vi "ChaxuConfigDlg.vi"(8 "error in":errorcluster) -> (0 "error out":errorcluster)   [LabVIEW 2014, in "ChaxuConfig.lvlib"]
uses:
  ChaxuConfig.lvlib
  <vilib>/Utility/file.llb/Write To Spreadsheet File (string).vi
  DataBase/DataBase.lvlib
  DetectElecrodes/DetectElectros.lvlib
panel:
  in  "表格导出":bool
  out "new file path (Not A Path if cancelled) 2":path caption="新建文件路径（取消时为非法路径）"
  in  "选项卡控件":enum32{"检测电极配置信息", "供电电极配置信息"}(tab)
  in  "配置信息":i32(listbox)
  in  "供电电极配置信息":i32(listbox)
  out "new file path (Not A Path if cancelled)":path caption="新建文件路径（取消时为非法路径）"
  in  "电极信息选择":u16(ring) items=["检测电极配置", "供电电极配置"]
  in  "表格导出":bool
  in  "查询":bool
  in  "退出":bool
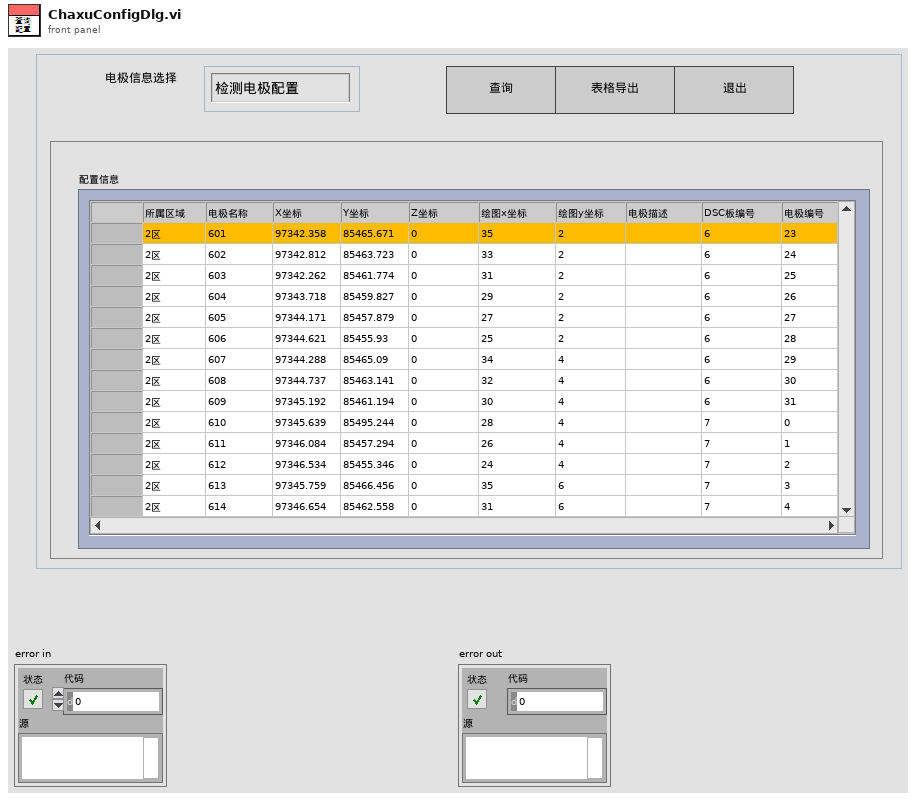
[diagram p1: front panel]
types:
  T1 = enum32{"invalid app kind", "Development System", "Run Time System", "Student Edition", "Embedded LabVIEW", "Evaluation", "Custom"}
  T2 = enum32{"Invalid", "Standard", "Closed", "Hidden", "Minimized", "Maximized"}
  T3 = cluster{"Core":cluster{"Current VI Reference":refnum<vi>, "Close Panel on Exit?":bool}, "Your Boolean data":bool, "Your string data":string, "电极信息":string[][]}
  T4 = cluster{"Current VI Reference":refnum<vi>, "Close Panel on Exit?":bool}
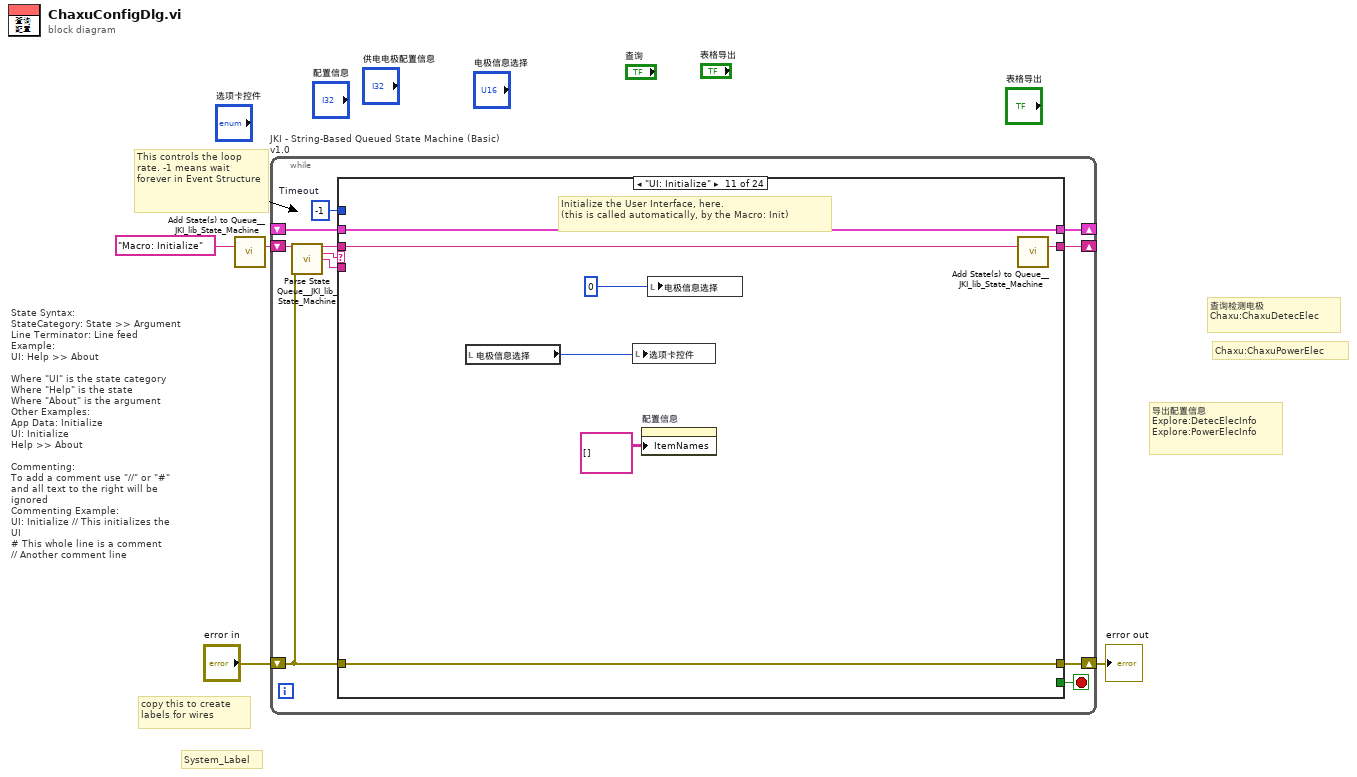
[diagram p0: block diagram]
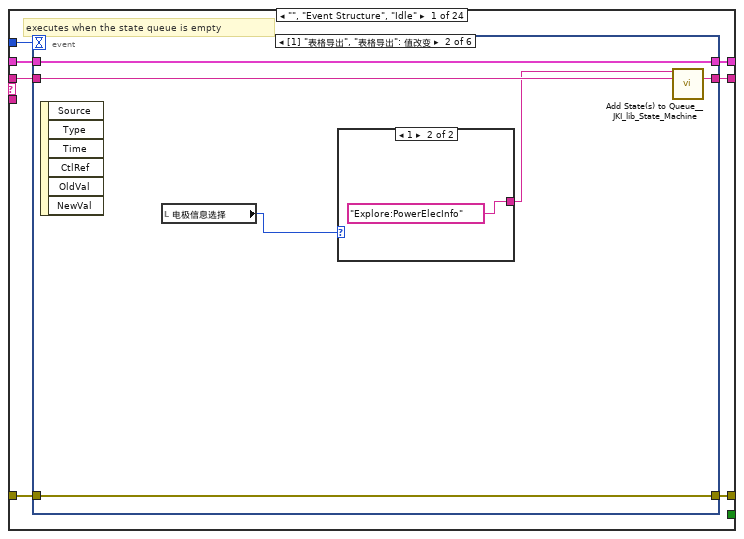
[diagram p2: hidden frame]
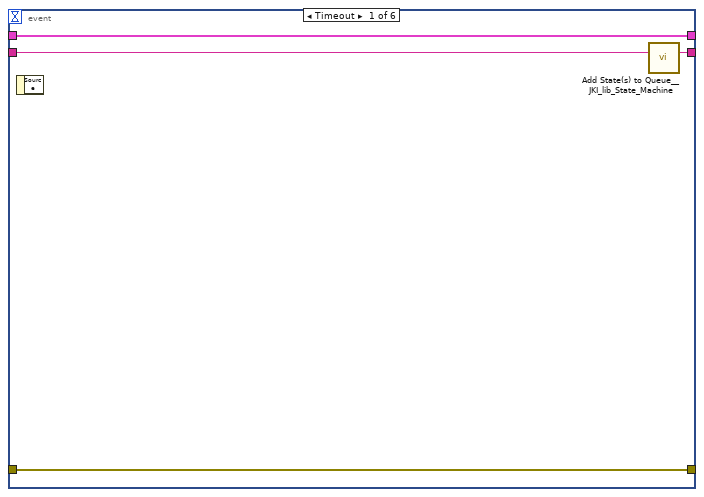
[diagram p3: hidden frame]
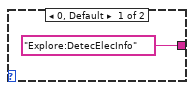
[diagram p4: hidden frame]
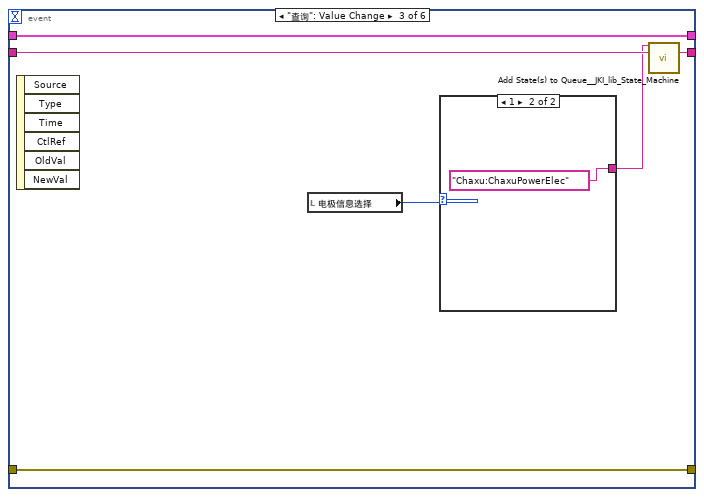
[diagram p5: hidden frame]
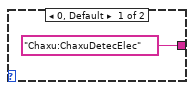
[diagram p6: hidden frame]
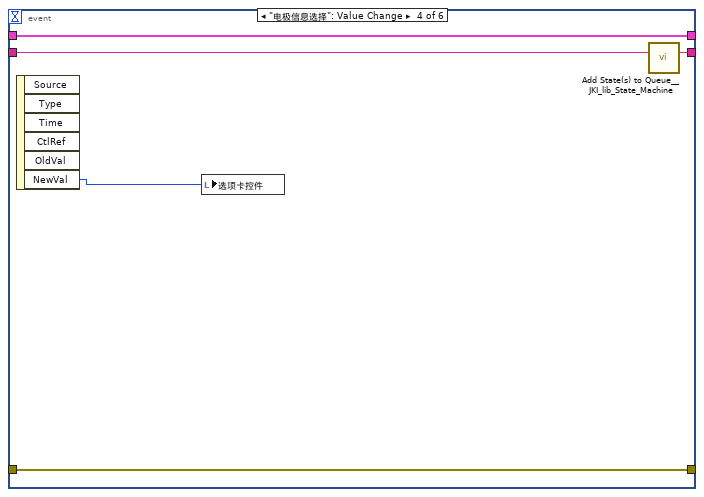
[diagram p7: hidden frame]
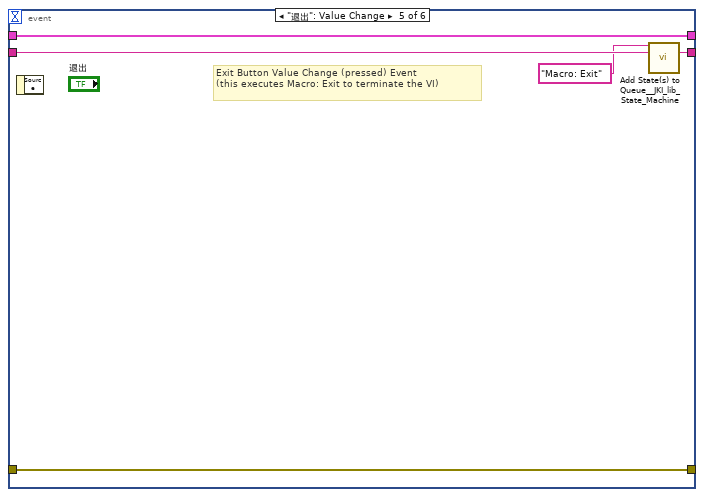
[diagram p8: hidden frame]
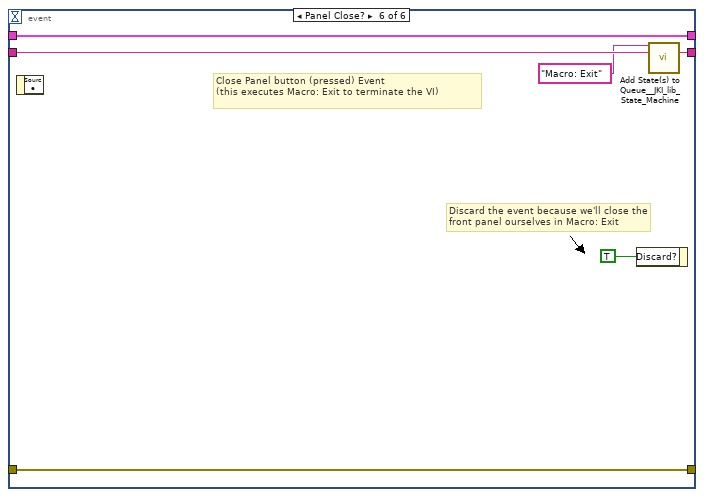
[diagram p9: hidden frame]
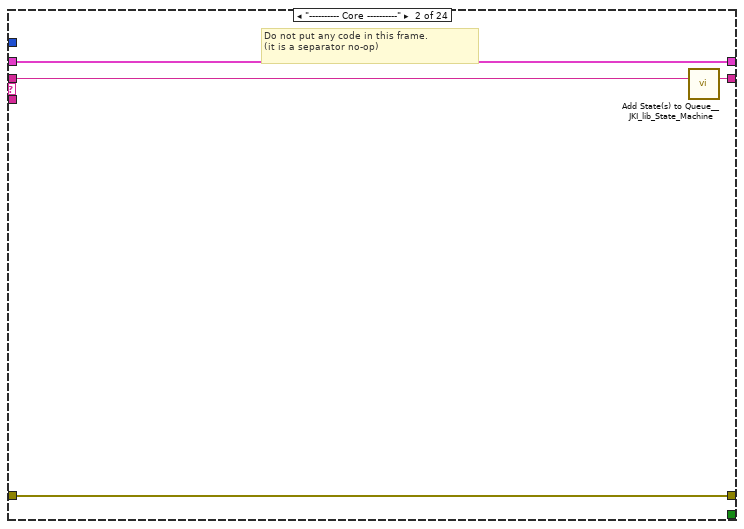
[diagram p10: hidden frame]
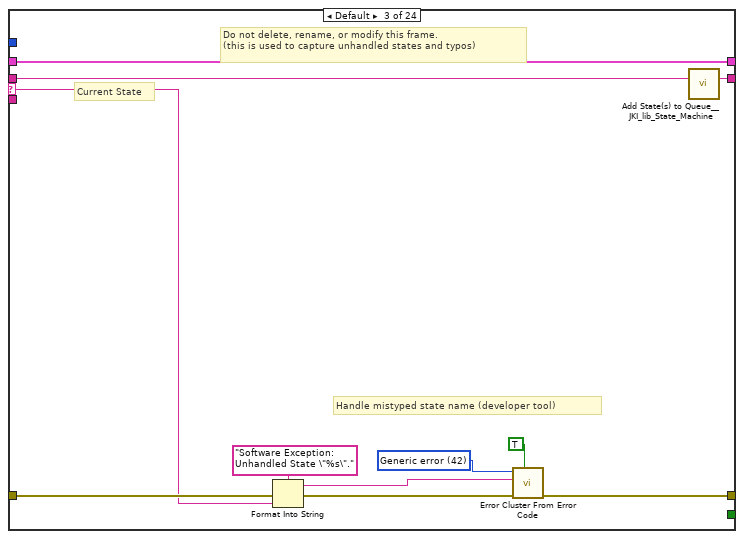
[diagram p11: hidden frame]
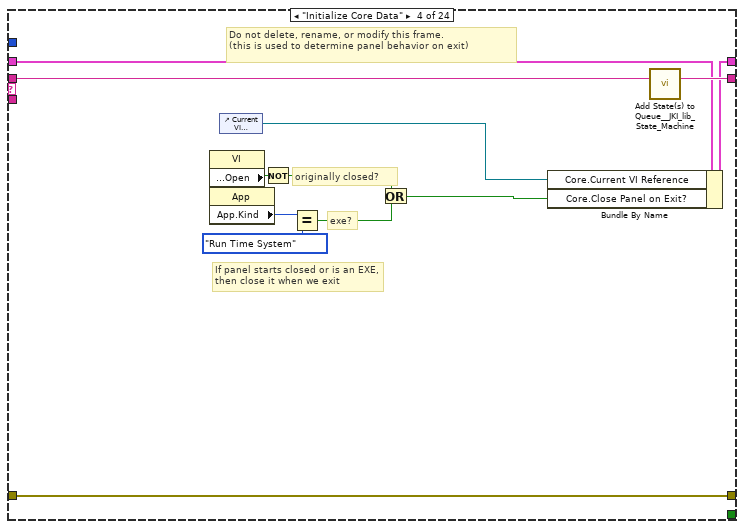
[diagram p12: hidden frame]
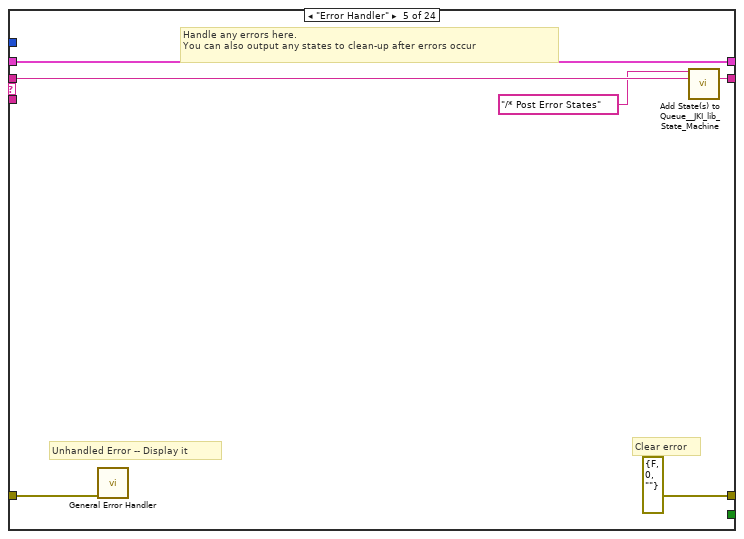
[diagram p13: hidden frame]
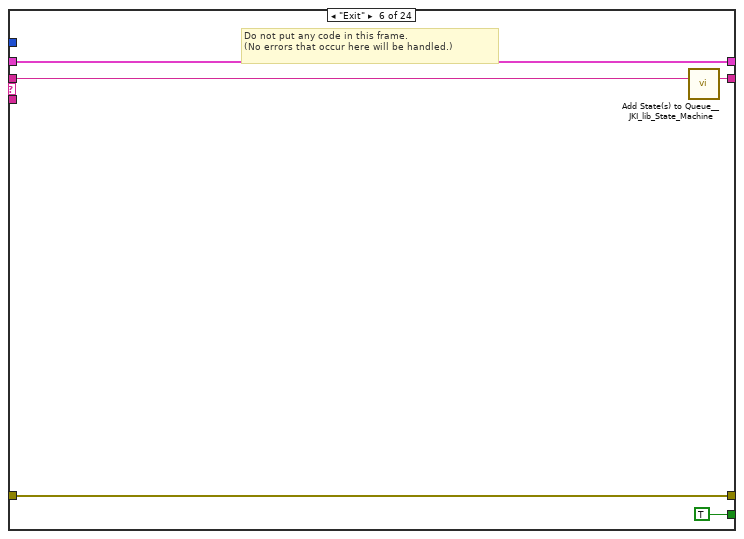
[diagram p14: hidden frame]
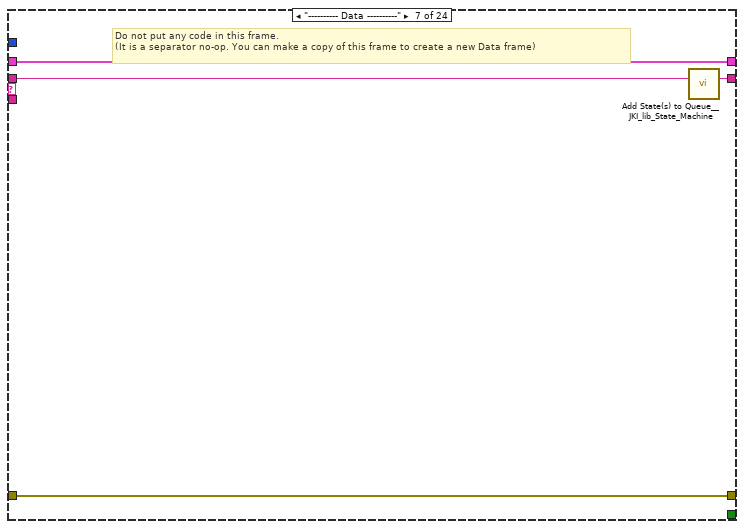
[diagram p15: hidden frame]
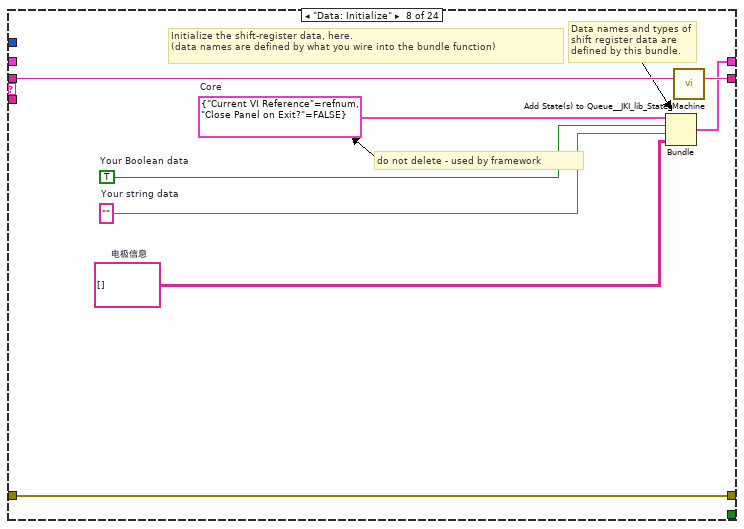
[diagram p16: hidden frame]
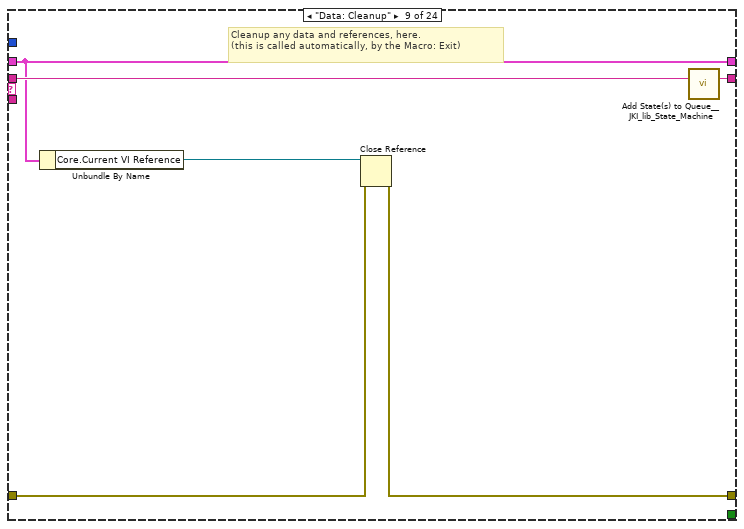
[diagram p17: hidden frame]
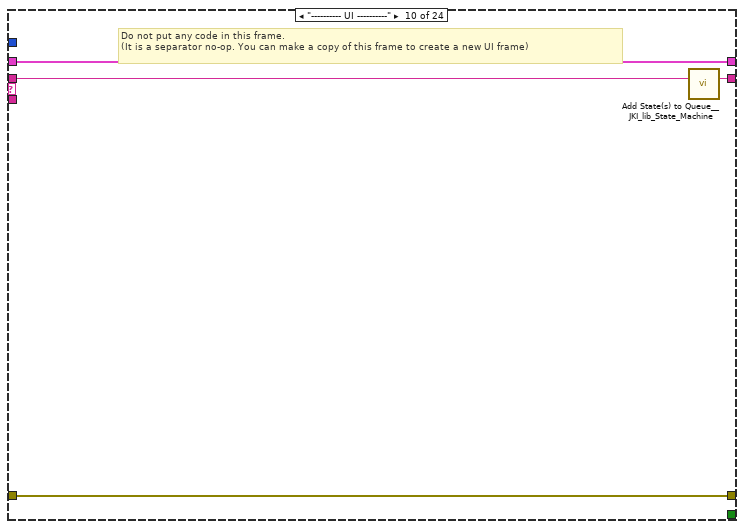
[diagram p18: hidden frame]
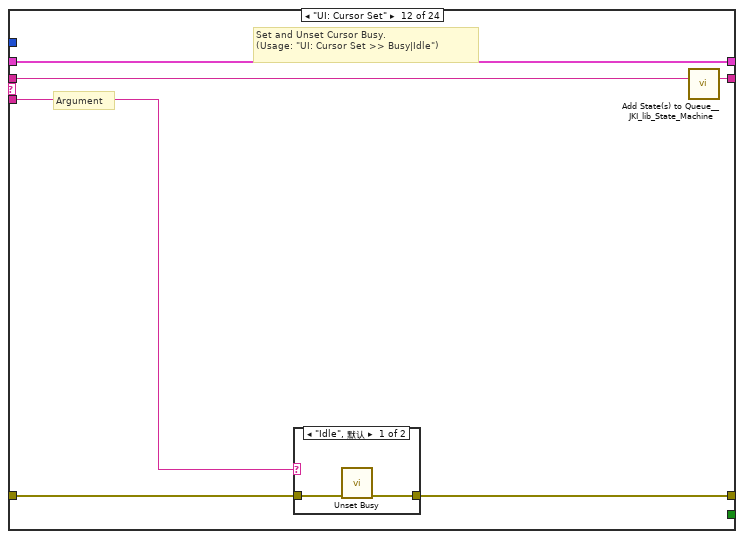
[diagram p19: hidden frame]
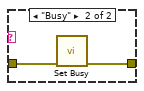
[diagram p20: hidden frame]
diagram:
  # "导出配置信息\nExplore:DetecElecInfo\nExplore:PowerElecInfo"
  # "Chaxu:ChaxuPowerElec"
  # "查询检测电极\nChaxu:ChaxuDetecElec"
  # "State Syntax:\nStateCategory: State >> Argument\nLine Terminator: Line feed\nExample:\nUI: Help >> About\n\nWhere \"UI\" is the state category\nWhere \"Help\" is the state\nWhere \"About\" is the argument\nOther Examples:\nApp Data: Initialize\nUI: Initialize\nHelp >> About\n\nCommenting:\nTo add a comment use \"//\" or \"#\" and all text to the right will be ignored\nCommenting Example:\nUI: Initialize // This initializes the UI\n# This whole line is a comment\n// Another comment line"
  # "copy this to create labels for wires"
  # "This controls the loop rate. -1 means wait forever in Event Structure"
  # "System_Label"
  n1 = call <vilib>:"Add State(s) to Queue__JKI_lib_State_Machine.vi"("State(s) in (\"\")"="Macro: Initialize") -> ("States Out"=w4:string)  [unwired: 14 in]
  n2 = while "JKI - String-Based Queued State Machine (Basic) v1.0" {
    shift-right: [w8] -> _
    shift-left: _ -> [w7]
    shift-right: [w11] -> w2
    shift-left: "error in" -> [w5]
    shift-right: [w10] -> _
    shift-left: w4 -> [w12]
    stop <- w9 stop-if-true
    w6 = -1  # Timeout
    n3 = call <vilib>:"Parse State Queue__JKI_lib_State_Machine.vi"("State Queue"=w12, "Error In (no error)"=w5) -> ("Remaining States"=w14:string, "Current State"=w15:string, "Arguments"=w13:string)  [unwired: 11 in]
    n4 = case shown="\"UI: Initialize\"" w15 {
      selector: w15 -> [_ _ w63 _ _ _ _ _ _ _ _ _ _ _ _ _ _ _ _ _ _ _ _ _]
      tunnel: w14 -> [w22 w62 w67 w85 w91 w96 w100 w108 w114 w118 w125 w131 w142 w168 w173 w183 w187 w191 w195 w200 w216 w231 w248 w265]
      tunnel: w13 -> [_ _ _ _ _ _ _ _ _ _ _ w126 w136 _ _ _ _ _ _ _ _ _ _ _]
      tunnel: w7 -> [w20 w59 w65 w76 w88 w94 w97 _ w109 w115 w123 w129 w138 w165 w170 w180 w184 w188 w192 w197 w213 w228 w233 w250]
      tunnel: [w19 w60 w69 w82 errorcluster {"status"=FALSE, "code"=0, "source"=""} ("error out") w93 w98 w105 w110 w116 w122 w127 w139 w166 w171 w181 w185 w189 w193 w198 w214 w229 w246 w263] -> w11
      tunnel: w5 -> [w18 w60 w68 w82 w87 w93 w98 w105 w111 w116 w122 w128 w140 w166 w171 w181 w185 w189 w193 w198 w214 w229 w246 w263]
      tunnel: [w21 w61 w66 w84 w90 w95 w99 w107 w113 w117 w124 w130 w141 w167 w172 w182 w186 w190 w194 w199 w215 w230 w247 w264] -> w10
      tunnel: [_ _ _ _ _ TRUE _ _ _ _ _ _ _ _ _ _ _ _ _ _ _ _ _ _] -> w9
      tunnel: [w17 w59 w65 w83 w88 w94 w97 w106 w109 w115 w123 w129 w138 w165 w170 w180 w184 w188 w192 w197 w213 w228 w232 w249] -> w8
      tunnel: w6 -> [w16 _ _ _ _ _ _ _ _ _ _ _ _ _ _ _ _ _ _ _ _ _ _ _]
      frame "", "Event Structure", "Idle" {
        # "executes when the state queue is empty"
        n5 = event shown="[1] \"表格导出\", \"表格导出\": 值改变" {
          selector: _ -> [_ _ _ _ _ _]
          dyn-events: _ -> [_ _ _ _ _ _]
          timeout: w16 -> [_ _ _ _ _ _]
          tunnel: w22 -> [w26 w32 w40 w47 w52 w58]
          tunnel: [w25 w31 w39 w46 w51 w57] -> w21
          tunnel: w20 -> [w23 w29 w37 w44 w49 w55]
          tunnel: [w24 w30 w38 w45 w50 w56] -> w19
          tunnel: w18 -> [w24 w30 w38 w45 w50 w56]
          tunnel: [w23 w29 w37 w44 w49 w55] -> w17
          event Timeout {
            n6 = event-data() -> ()  [unwired: 1 in, 1 out]
            n7 = call <vilib>:"Add State(s) to Queue__JKI_lib_State_Machine.vi"("State(s) in (\"\")"=w26) -> ("States Out"=w25:string)  [unwired: 14 in]
          }
          event "表格导出", "表格导出": Value Change {
            n8 = event-data() -> ()  [unwired: 1 in, 6 out]
            n9 = local read "电极信息选择"() -> (w27:u16)
            n10 = case shown="1" w27 {
              tunnel: ["Explore:DetecElecInfo" "Explore:PowerElecInfo"] -> w28
              frame 0, Default {
              }
              frame 1 {
              }
            }
            n11 = call <vilib>:"Add State(s) to Queue__JKI_lib_State_Machine.vi"("State(s) in Front (\"\")"=w28, "State(s) in (\"\")"=w32) -> ("States Out"=w31:string)  [unwired: 13 in]
          }
          event "查询": Value Change {
            n12 = event-data() -> ()  [unwired: 1 in, 6 out]
            n13 = local read "电极信息选择"() -> (w36:u16)
            n14 = case shown="1" w36 {
              tunnel: ["Chaxu:ChaxuDetecElec" "Chaxu:ChaxuPowerElec"] -> w35
              frame 0, Default {
              }
              frame 1 {
              }
            }
            n15 = call <vilib>:"Add State(s) to Queue__JKI_lib_State_Machine.vi"("State(s) in Front (\"\")"=w35, "State(s) in (\"\")"=w40) -> ("States Out"=w39:string)  [unwired: 13 in]
          }
          event "电极信息选择": Value Change {
            n16 = event-data() -> ("NewVal"=w43:u16)  [unwired: 1 in, 5 out]
            n17 = local write "选项卡控件"(w43) -> ()
            n18 = call <vilib>:"Add State(s) to Queue__JKI_lib_State_Machine.vi"("State(s) in (\"\")"=w47) -> ("States Out"=w46:string)  [unwired: 14 in]
          }
          event "退出": Value Change {
            # "Exit Button Value Change (pressed) Event\n(this executes Macro: Exit to terminate the VI)"
            n19 = event-data() -> ()  [unwired: 1 in, 1 out]
            n20 = call <vilib>:"Add State(s) to Queue__JKI_lib_State_Machine.vi"("State(s) in Front (\"\")"="Macro: Exit", "State(s) in (\"\")"=w52) -> ("States Out"=w51:string)  [unwired: 13 in]
          }
          event Panel Close? {
            # "Discard the event because we'll close the front panel ourselves in Macro: Exit"
            # "Close Panel button (pressed) Event\n(this executes Macro: Exit to terminate the VI)"
            n21 = event-data() -> ()  [unwired: 1 in, 1 out]
            n22 = event-data("Discard?"=TRUE) -> ()  [unwired: 1 in, 1 out]
            n23 = call <vilib>:"Add State(s) to Queue__JKI_lib_State_Machine.vi"("State(s) in Front (\"\")"="Macro: Exit", "State(s) in (\"\")"=w58) -> ("States Out"=w57:string)  [unwired: 13 in]
          }
        }
      }
      frame "---------- Core ----------" {
        # "Do not put any code in this frame.\n(it is a separator no-op)"
        n24 = call <vilib>:"Add State(s) to Queue__JKI_lib_State_Machine.vi"("State(s) in (\"\")"=w62) -> ("States Out"=w61:string)  [unwired: 14 in]
      }
      frame Default {
        w72 = 42 items=["No error", "Argument error", "Memory is full", "Out of zone", "End of file", "File already open", "Generic file I/O error", "File not found", "File permission error", "Disk is full", "Duplicate path", "Too many files open", "System feature not enabled", "Resource file not found", "Cannot add resource", "Resource not found", "Image not found", "Image memory error", "Pen does not exist", "Config type invalid", "Config token not found", "Config parse error", "Config memory error", "Bad external code format", "Bad external code offset", "External code not present", "Null window", "Destroy window error", "Null menu", "Print aborted", "Bad print record", "Print driver error", "Windows error during printing", "Memory error during printing", "Print dialog error", "Generic print error", "Invalid device refnum", "Device not found", "Device parameter error", "Device unit error", "Cannot open device", "Device call aborted", "Generic error", "Cancelled by user", "Object ID too low", "Object ID too high", "Object not in heap", "Unknown heap", "Unknown object (invalid DefProc)", "Unknown object (DefProc not in table)", "Message out of range", "Invalid (null) method", "Unknown message", "Manager call not supported", "Bad address", "Network operation in progress", "Network operation timed out", "Connection is busy", "Network attribute not supported", "Network error", "Address in use", "System out of memory", "Connection aborted", "Connection refused", "Not connected", "Already connected", "Connection closed", "Initialization error (interapplication manager)", "Bad occurrence", "Wait on unbound occurrence handler", "Occurrence queue overflow", "Datalog type conflict", "Unused", "Unrecognized type (interapplication manager)", "Memory corrupt", "Failed to make temporary DLL", "Old CIN version", "Drag socket not found", "Failed to load drop-object", "Failed to register OLE object", "Failed to release OLE object", "Format specifier type mismatch", "Unknown format specifier", "Too few format specifiers", "Too many format specifiers", "Scan failed", "Newer CIN version", "Error converting to variant", "Runtime menu error", "Password tampered", "Variant attribute not found", "Incompatible variant data type", "Event data is not available", "Event Store is not present", "Occurrence is not found", "Event Queue is not created", "Event info is not available", "Refnum passed is NULL", "Error retrieving Class GUID", "Error retrieving CoClass GUID", "Error retrieving TypeLib GUID.", "Bad built application magic bytes.", "Specific driver is different from the specific driver associated with the Logical Name.", "There is no session opened to the class driver.", "Max Error", "MAX - Error with config objects", "MAX - Error loading configuration", "MAX - Group not supported"]
        # "Current State"
        # "Do not delete, rename, or modify this frame.\n(this is used to capture unhandled states and typos)"
        # "Handle mistyped state name (developer tool)"
        n25 = Format Into String(format string="Software Exception: Unhandled State \"%s\"." ("message"), error in=w68, w63) -> (resulting string=w71:string, error out=w70:errorcluster)  [unwired: 1 in]
        n26 = call <vilib>:"Error Cluster From Error Code.vi"("show call chain? (False)"=TRUE, "error in (no error)"=w70, "error message (\"\")"=w71, "error code (0)"=w72) -> ("error out"=w69:errorcluster)  [unwired: 5 in]
        n27 = call <vilib>:"Add State(s) to Queue__JKI_lib_State_Machine.vi"("State(s) in (\"\")"=w67) -> ("States Out"=w66:string)  [unwired: 14 in]
      }
      frame "Initialize Core Data" {
        # "Do not delete, rename, or modify this frame.\n(this is used to determine panel behavior on exit)"
        # "originally closed?"
        # "exe?"
        # "If panel starts closed or is an EXE, then close it when we exit"
        n28 = property class="VI"() -> ("Front Panel.Open"=w81:bool)  [unwired: 2 in, 2 out]
        n29 = property class="App"() -> ("App.Kind"=w80:T1)  [unwired: 2 in, 2 out]
        n30 = control-ref of="Current VI Reference"() -> (w74:refnum<vi>)
        n31 = Not(x=w81) -> (.not. x?=w78:bool)
        n32 = Equal?(x=w80, y=T1."Run Time System" ("Application:Kind")) -> (x = y?=w77:bool)
        n33 = Or(x=w78, y=w77) -> (x .or. y?=w75:bool)
        n34 = Bundle By Name(cluster=w76, "Core.Current VI Reference"=w74, "Core.Close Panel on Exit?"=w75) -> (w83:T3)
        n35 = call <vilib>:"Add State(s) to Queue__JKI_lib_State_Machine.vi"("State(s) in (\"\")"=w85) -> ("States Out"=w84:string)  [unwired: 14 in]
      }
      frame "Error Handler" {
        # "Unhandled Error -- Display it"
        # "Handle any errors here.\nYou can also output any states to clean-up after errors occur"
        # "Clear error"
        n36 = call <vilib>:"General Error Handler.vi"("error in (no error)"=w87) -> ()  [unwired: 10 in, 5 out]
        n37 = call <vilib>:"Add State(s) to Queue__JKI_lib_State_Machine.vi"("State(s) in Front (\"\")"="/* Post Error States", "State(s) in (\"\")"=w91) -> ("States Out"=w90:string)  [unwired: 13 in]
      }
      frame "Exit" {
        # "Do not put any code in this frame.\n(No errors that occur here will be handled.)"
        n38 = call <vilib>:"Add State(s) to Queue__JKI_lib_State_Machine.vi"("State(s) in (\"\")"=w96) -> ("States Out"=w95:string)  [unwired: 14 in]
      }
      frame "---------- Data ----------" {
        # "Do not put any code in this frame.\n(It is a separator no-op. You can make a copy of this frame to create a new Data frame)"
        n39 = call <vilib>:"Add State(s) to Queue__JKI_lib_State_Machine.vi"("State(s) in (\"\")"=w100) -> ("States Out"=w99:string)  [unwired: 14 in]
      }
      frame "Data: Initialize" {
        w101 = string[][] []  # 电极信息
        w102 = T4 {"Current VI Reference"=refnum, "Close Panel on Exit?"=FALSE}  # Core
        w104 = TRUE  # Your Boolean data
        w103 = ""  # Your string data
        # "do not delete - used by framework"
        # "Data names and types of shift register data are defined by this bundle."
        # "Initialize the shift-register data, here.\n(data names are defined by what you wire into the bundle function)"
        n40 = Bundle("Core"=w102, "Your Boolean data"=w104, "Your string data"=w103, "电极信息"=w101) -> (w106:T3)  [unwired: 1 in]
        n41 = call <vilib>:"Add State(s) to Queue__JKI_lib_State_Machine.vi"("State(s) in (\"\")"=w108) -> ("States Out"=w107:string)  [unwired: 14 in]
      }
      frame "Data: Cleanup" {
        # "Cleanup any data and references, here.\n(this is called automatically, by the Macro: Exit)"
        n42 = Unbundle By Name(w109) -> ("Core.Current VI Reference"=w112:refnum<vi>)
        n43 = Close Reference(reference=w112, error in (no error)=w111) -> (error out=w110:errorcluster)
        n44 = call <vilib>:"Add State(s) to Queue__JKI_lib_State_Machine.vi"("State(s) in (\"\")"=w114) -> ("States Out"=w113:string)  [unwired: 14 in]
      }
      frame "---------- UI ----------" {
        # "Do not put any code in this frame.\n(It is a separator no-op. You can make a copy of this frame to create a new UI frame)"
        n45 = call <vilib>:"Add State(s) to Queue__JKI_lib_State_Machine.vi"("State(s) in (\"\")"=w118) -> ("States Out"=w117:string)  [unwired: 14 in]
      }
      frame "UI: Initialize" {
        # "Initialize the User Interface, here.\n(this is called automatically, by the Macro: Init)"
        n46 = local read "电极信息选择"() -> (w121:u16)
        n47 = local write "选项卡控件"(w121) -> ()
        n48 = property on="配置信息" class="MCListbox (严格)"("ItemNames"=string[][] [] ("项名")) -> ()  [unwired: 2 in, 2 out]
        n49 = local write "电极信息选择"(0) -> ()
        n50 = call <vilib>:"Add State(s) to Queue__JKI_lib_State_Machine.vi"("State(s) in (\"\")"=w125) -> ("States Out"=w124:string)  [unwired: 14 in]
      }
      frame "UI: Cursor Set" {
        # "Argument"
        # "Set and Unset Cursor Busy.\n(Usage: \"UI: Cursor Set >> Busy|Idle\")"
        n51 = case shown="\"Idle\", 默认" w126 {
          tunnel: w128 -> [w133 w135]
          tunnel: [w132 w134] -> w127
          frame "Idle", Default {
            n52 = call <vilib>:"Unset Busy.vi"("error in (no error)"=w133) -> ("error out"=w132:errorcluster)  [unwired: 10 in]
          }
          frame "Busy" {
            n53 = call <vilib>:"Set Busy.vi"("error in (no error)"=w135) -> ("error out"=w134:errorcluster)  [unwired: 9 in, 1 out]
          }
        }
        n54 = call <vilib>:"Add State(s) to Queue__JKI_lib_State_Machine.vi"("State(s) in (\"\")"=w131) -> ("States Out"=w130:string)  [unwired: 14 in]
      }
      frame "UI: Front Panel State" {
        # "Argument"
        # "Set Front Panel Open or Closed\n(Usage: \"UI: Front Panel State >> Open|Close\")"
        n55 = Unbundle By Name(w138) -> ("Core.Current VI Reference"=w137:refnum<vi>)
        n56 = case shown="\"Open\", 默认" w136 {
          tunnel: w140 -> [w146 w159]
          tunnel: [w148 w160] -> w139
          tunnel: w137 -> [w147 w157]
          frame "Open", Default {
            n57 = property class="VI"(reference=w147, error in=w146) -> (reference out=w144:refnum<vi>, error out=w145:errorcluster, "Front Panel.Open"=w143:bool)
            n58 = case shown="假" w143 {
              tunnel: [w151 w154] -> w148
              tunnel: w145 -> [w150 w154]
              tunnel: w144 -> [w149 _]
              frame False {
                n59 = invoke class="VI" method="FP.Open"(reference=w149, error in=w150, "Activate"=TRUE, "State"=T2."Standard") -> (error out=w151:errorcluster)  [unwired: 1 in, 4 out]
              }
              frame True {
              }
            }
          }
          frame "Close" {
            n60 = property class="VI"(reference=w157, error in=w159) -> (reference out=w156:refnum<vi>, error out=w158:errorcluster, "Front Panel.Open"=w155:bool)
            n61 = case shown="真" w155 {
              tunnel: [w161 w164] -> w160
              tunnel: w158 -> [w161 w163]
              tunnel: w156 -> [_ w162]
              frame False {
              }
              frame True {
                n62 = invoke class="VI" method="FP.Close"(reference=w162, error in=w163) -> (error out=w164:errorcluster)  [unwired: 1 in, 2 out]
              }
            }
          }
        }
        n63 = call <vilib>:"Add State(s) to Queue__JKI_lib_State_Machine.vi"("State(s) in (\"\")"=w142) -> ("States Out"=w141:string)  [unwired: 14 in]
      }
      frame "---------- Macro ----------" {
        # "Do not put any code in this frame.\n(It is a separator no-op. You can make a copy of this frame to create a new Macro frame)"
        n64 = call <vilib>:"Add State(s) to Queue__JKI_lib_State_Machine.vi"("State(s) in (\"\")"=w168) -> ("States Out"=w167:string)  [unwired: 14 in]
      }
      frame "Macro: Initialize" {
        w169 = "Data: Initialize\nInitialize Core Data\nUI: Initialize\nUI: Front Panel State >> Open"  # Data: Initialize Initialize Core Data UI: Initialize UI: Front Panel State >> Open
        # "Initialization Macro\n(This is called once, when the VI starts)"
        n65 = call <vilib>:"Add State(s) to Queue__JKI_lib_State_Machine.vi"("State(s) in Front (\"\")"=w169, "State(s) in (\"\")"=w173) -> ("States Out"=w172:string)  [unwired: 13 in]
      }
      frame "Macro: Exit" {
        # "Exit Macro\n(This is called once, when the VI exits)"
        n66 = Unbundle By Name(w180) -> ("Core.Close Panel on Exit?"=w179:bool)
        n67 = Select(t="UI: Front Panel State >> Close", s=w179, f="") -> (s? t:f=w176:string)
        n68 = call <vilib>:"Add State(s) to Queue__JKI_lib_State_Machine.vi"("State(s) in (\"\")"=w176, "State(s) at Back (\"\")"="Data: Cleanup\nExit") -> ("States Out"=w174:string)  [unwired: 13 in]
        n69 = call <vilib>:"Add State(s) to Queue__JKI_lib_State_Machine.vi"("State(s) in Front (\"\")"=w174, "State(s) in (\"\")"=w183) -> ("States Out"=w182:string)  [unwired: 13 in]
      }
      frame "---------- New Category ----------" {
        # "Template Separator\n(You can make a copy of, or modify, this frame)"
        n70 = call <vilib>:"Add State(s) to Queue__JKI_lib_State_Machine.vi"("State(s) in (\"\")"=w187) -> ("States Out"=w186:string)  [unwired: 14 in]
      }
      frame "New Category: 1" {
        # "Your code here.\n(You can make a copy of, or modify, this frame)"
        n71 = call <vilib>:"Add State(s) to Queue__JKI_lib_State_Machine.vi"("State(s) in (\"\")"=w191) -> ("States Out"=w190:string)  [unwired: 14 in]
      }
      frame "New Category: 2" {
        # "Your code here.\n(You can make a copy of, or modify, this frame)"
        n72 = call <vilib>:"Add State(s) to Queue__JKI_lib_State_Machine.vi"("State(s) in (\"\")"=w195) -> ("States Out"=w194:string)  [unwired: 14 in]
      }
      frame "Explore:DetecElecInfo" {
        n73 = flat-sequence {
          tunnel: w197 -> [w210]
          tunnel: ["电极配置导出成功"] -> w196
          tunnel: w196 -> [w211]
          frame #0 {
            n74 = property on="配置信息" class="MCListbox (严格)"() -> ("ColHdrString"=w204:string[])  [unwired: 2 in, 2 out]
            n75 = Unbundle By Name(w210) -> ("电极信息"=w207:string[][])
            n76 = call "SavePath.vi"("字符串"="采样电极配置") -> ("appended path"=w202:path)  [unwired: 10 in]
            n77 = Insert Into Array(array=w207, index (row)=0 ("索引 (行)"), new element=w204) -> (w205:string[][])  [unwired: 1 in]
            n78 = call-poly <vilib>:"Write To Spreadsheet File.vi"("delimiter (\\t)"="," ("delimiter (\\t)"), "2D data"=w205, "file path (dialog if empty)"=w202) -> ("new file path (Not A Path if cancelled)"=→"new file path (Not A Path if cancelled)":path)  [unwired: 5 in]
          }
          frame #1 {
            n79 = One Button Dialog(message=w211) -> ()  [unwired: 1 in, 1 out]
          }
        }
        n80 = call <vilib>:"Add State(s) to Queue__JKI_lib_State_Machine.vi"("State(s) in (\"\")"=w200) -> ("States Out"=w199:string)  [unwired: 14 in]
      }
      frame "Explore:PowerElecInfo" {
        n81 = flat-sequence {
          tunnel: w213 -> [w226]
          tunnel: ["供电电极配置成功"] -> w212
          tunnel: w212 -> [w227]
          frame #0 {
            n82 = property on="供电电极配置信息" class="MCListbox (严格)"() -> ("ColHdrString"=w220:string[])  [unwired: 2 in, 2 out]
            n83 = Unbundle By Name(w226) -> ("电极信息"=w223:string[][])
            n84 = call "SavePath.vi"("字符串"="供电电极配置") -> ("appended path"=w218:path)  [unwired: 10 in]
            n85 = Insert Into Array(array=w223, index (row)=0 ("索引 (行)"), new element=w220) -> (w221:string[][])  [unwired: 1 in]
            n86 = call-poly <vilib>:"Write To Spreadsheet File.vi"("delimiter (\\t)"="," ("delimiter (\\t)"), "2D data"=w221, "file path (dialog if empty)"=w218) -> ("new file path (Not A Path if cancelled)"=→"new file path (Not A Path if cancelled) 2":path)  [unwired: 5 in]
          }
          frame #1 {
            n87 = One Button Dialog(message=w227) -> ()  [unwired: 1 in, 1 out]
          }
        }
        n88 = call <vilib>:"Add State(s) to Queue__JKI_lib_State_Machine.vi"("State(s) in (\"\")"=w216) -> ("States Out"=w215:string)  [unwired: 14 in]
      }
      frame "---------Chaxu----------" {
        # "Your code here.\n(You can make a copy of, or modify, this frame)"
        n89 = call <vilib>:"Add State(s) to Queue__JKI_lib_State_Machine.vi"("State(s) in (\"\")"=w231) -> ("States Out"=w230:string)  [unwired: 14 in]
      }
      frame "Chaxu:ChaxuDetecElec" {
        n90 = call "SelectData.vi"("SQL query"="select * from t_detection_electrodes;") -> ("recordset data"=w244:variant[][])  [unwired: 7 in, 1 out]
        n91 = call "ReadDataFromDatabase.vi"("长度"=11, "index"=1, "recordset data"=w244) -> ("所有记录"=w238:string[][])  [unwired: 7 in, 1 out]
        n92 = Array Subset(array=w238, index (col)=0, length (col)=1 ("长度")) -> (w236:string[][])  [unwired: 2 in]
        n93 = Array Subset(array=w238, index (col)=1) -> (w235:string[][])  [unwired: 3 in]
        n94 = Insert Into Array(array=w235, index (col)=1 ("禁用的索引 (列)"), new element=w236) -> (w234:string[][])  [unwired: 1 in]
        n95 = Bundle By Name(cluster=w233, "电极信息"=w234) -> (w232:T3)
        n96 = property on="配置信息" class="MCListbox (严格)"("ItemNames"=w234) -> ()  [unwired: 2 in, 2 out]
        n97 = call <vilib>:"Add State(s) to Queue__JKI_lib_State_Machine.vi"("State(s) in (\"\")"=w248) -> ("States Out"=w247:string)  [unwired: 14 in]
      }
      frame "Chaxu:ChaxuPowerElec" {
        n98 = call "SelectData.vi"("SQL query"="select * from t_power_electrodes;") -> ("recordset data"=w261:variant[][])  [unwired: 7 in, 1 out]
        n99 = call "ReadDataFromDatabase.vi"("长度"=9, "index"=1, "recordset data"=w261) -> ("所有记录"=w256:string[][])  [unwired: 7 in, 1 out]
        n100 = Array Subset(array=w256, index (col)=0 ("索引"), length (col)=1 ("长度")) -> (w253:string[][])  [unwired: 2 in]
        n101 = Array Subset(array=w256, index (col)=1 ("索引")) -> (w254:string[][])  [unwired: 3 in]
        n102 = Insert Into Array(array=w254, index (col)=1 ("禁用的索引 (列)"), new element=w253) -> (w251:string[][])  [unwired: 1 in]
        n103 = Bundle By Name(cluster=w250, "电极信息"=w251) -> (w249:T3)
        n104 = property on="供电电极配置信息" class="MCListbox (严格)"("ItemNames"=w251) -> ()  [unwired: 2 in, 2 out]
        n105 = call <vilib>:"Add State(s) to Queue__JKI_lib_State_Machine.vi"("State(s) in (\"\")"=w265) -> ("States Out"=w264:string)  [unwired: 14 in]
      }
    }
  }
  "error out" <- w2
